vi "FSK_Convcode.vi"(8 "error in (no error)":errorcluster caption="错误输入（无错误）", 10 "input_data":dbl[](array[numeric]), 11 "PathIn":path) -> (0 "error out":errorcluster caption="错误输出", 2 "output_data":dbl[](array[numeric]) format="%#_13g", 3 "PathOut":path)   [LabVIEW 2015]
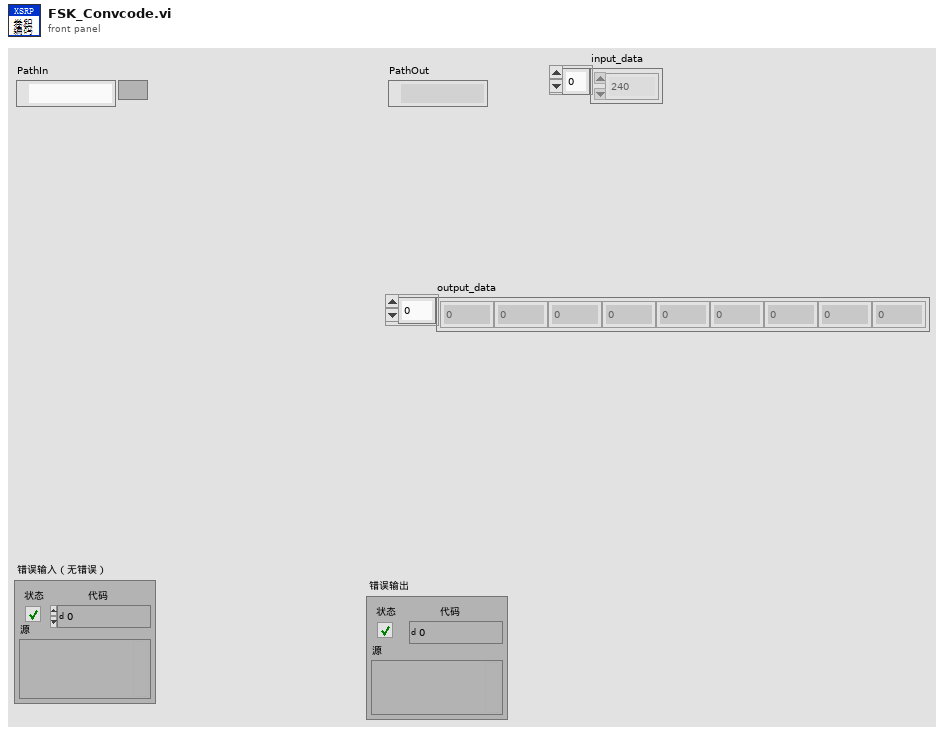
[diagram p1: front panel]
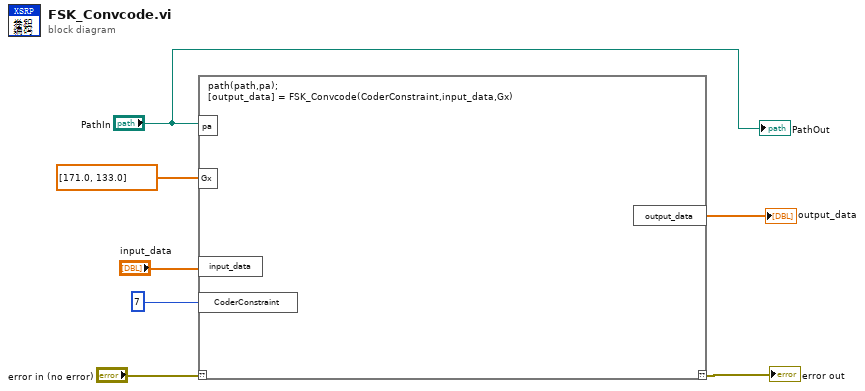
[diagram p0: block diagram]
diagram:
  n1 = script code="path(path,pa);\n[output_data] = FSK_Convcode(CoderConstraint,input_data,Gx)"("??"="error in (no error)", "pa"="PathIn", "input_data"="input_data", "CoderConstraint"=7, "Gx"=dbl[] [171.0, 133.0]) -> ("??"=→"error out":errorcluster, "output_data"=→"output_data":dbl[])
  "PathOut" <- "PathIn"
